vi "LV_parser.vi"(0 "Open .lv file":path) -> (1 "Track Array":i32[][][](array[numeric]), 2 "Starting array":dbl[](array[numeric]))   [LabVIEW 2012]
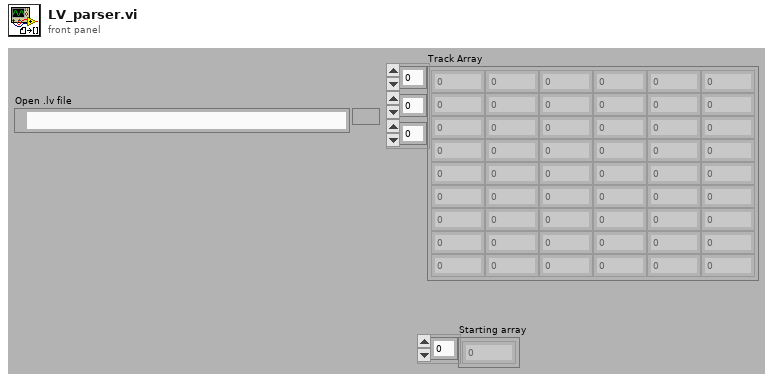
[diagram p1: front panel]
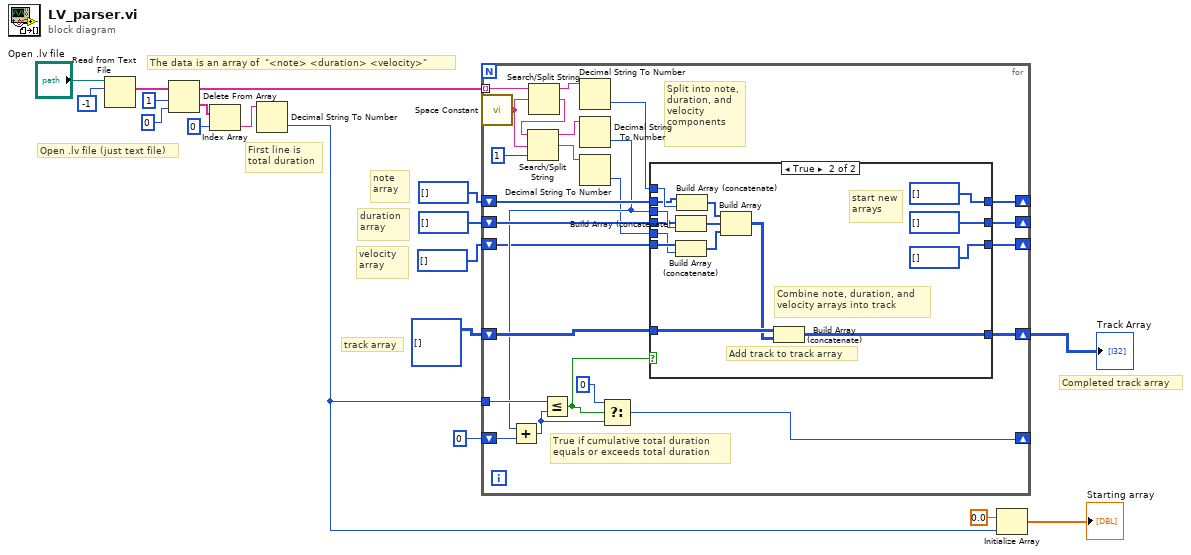
[diagram p0: block diagram]
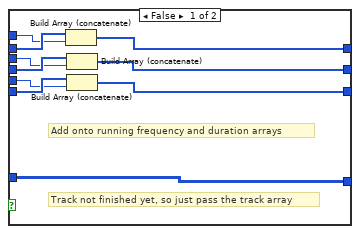
[diagram p2: hidden frame]
diagram:
  # "velocity array"
  # "Completed track array"
  # "track array"
  # "duration array"
  # "note array"
  # "The data is an array of  \"<note> <duration> <velocity>\""
  # "First line is total duration"
  # "Open .lv file (just text file)"
  n1 = Read from Text File(file (use dialog)="Open .lv file", count=-1) -> (text=w16:string[])  [unwired: 2 in, 3 out]
  n2 = Delete From Array(array=w16, length=1, index=0) -> (deleted portion=w13:string[], array with subset deleted=w9:string[])
  n3 = Index Array(array=w13, index=0) -> (element=w11:string)
  n4 = Decimal String To Number(string=w11) -> (number=w3:i32)  [unwired: 2 in, 1 out]
  n5 = for {
    tunnel: w3 -> [w40]
    shift-right: [w42] -> _
    shift-left: 0 -> [w29]
    tunnel: w9 -> [w39] mode=indexing
    shift-right: [w33] -> _
    shift-left: i32[] [] -> [w35]
    shift-right: [w31] -> w5
    shift-left: i32[][][] [] -> [w32]
    shift-right: [w34] -> _
    shift-left: i32[] [] -> [w36]
    shift-right: [w22] -> _
    shift-left: i32[] [] -> [w24]
    # "True if cumulative total duration equals or exceeds total duration"
    # "Split into note,  duration, and velocity components"
    n6 = call <vilib>:"Space Constant.vi"() -> ("String"=w21:string)
    n7 = Search/Split String(string=w39, search string/char (-)=w21) -> (substring before match=w38:string, match + rest of string=w27:string)  [unwired: 1 in, 1 out]
    n8 = Search/Split String(string=w27, search string/char (-)=w21, offset (0)=1) -> (substring before match=w26:string, match + rest of string=w25:string)  [unwired: 1 out]
    n9 = Decimal String To Number(string=w38) -> (number=w19:i32)  [unwired: 2 in, 1 out]
    n10 = Decimal String To Number(string=w26) -> (number=w30:i32)  [unwired: 2 in, 1 out]
    n11 = Add(x=w30, y=w29) -> (x+y=w28:i32)
    n12 = Less Or Equal?(x=w40, y=w28) -> (x <= y?=w37:bool)
    n13 = Decimal String To Number(string=w25) -> (number=w23:i32)  [unwired: 2 in, 1 out]
    n14 = Select(t=0, s=w37, f=w28) -> (s? t:f=w42:i32)
    n15 = case shown="True" w37 {
      tunnel: w36 -> [w52 w64]
      tunnel: w35 -> [w49 w62]
      tunnel: [w50 i32[] []] -> w34
      tunnel: [w47 i32[] []] -> w33
      tunnel: w19 -> [w51 w65]
      tunnel: w30 -> [w48 w63]
      tunnel: w32 -> [w46 w61]
      tunnel: [w46 w60] -> w31
      tunnel: w24 -> [w45 w59]
      tunnel: w23 -> [w43 w58]
      tunnel: [w44 i32[] []] -> w22
      frame False {
        # "Track not finished yet, so just pass the track array"
        # "Add onto running frequency and duration arrays"
        n16 = Build Array (concatenate)(w52, w51) -> (w50:i32[])
        n17 = Build Array (concatenate)(w49, w48) -> (w47:i32[])
        n18 = Build Array (concatenate)(w45, w43) -> (w44:i32[])
      }
      frame True {
        # "Combine note, duration, and velocity arrays into track"
        # "Add track to track array"
        # "start new arrays"
        n19 = Build Array (concatenate)(w62, w63) -> (w55:i32[])
        n20 = Build Array (concatenate)(w59, w58) -> (w54:i32[])
        n21 = Build Array (concatenate)(w64, w65) -> (w56:i32[])
        n22 = Build Array(w56, w55, w54) -> (w53:i32[][])
        n23 = Build Array (concatenate)(w61, w53) -> (w60:i32[][][])
      }
    }
  }
  "Track Array" <- w5
  n24 = Initialize Array(0.0 ("element"), w3) -> (→"Starting array":dbl[])
